vi "Create Instrument SMO Name.vi"(8 "error in (no error)":errorcluster, 11 "Instrument.Lockin":refnum<class "Instrument.Lockin.lvclass">) -> (0 "error out":errorcluster, 2 "SMO Name":string, 3 "Instrument.Lockin out":refnum<class "Instrument.Lockin.lvclass">)   [LabVIEW 2016, in "Instrument.Lockin.lvclass"]
uses:
  Instrument.Lockin.lvclass
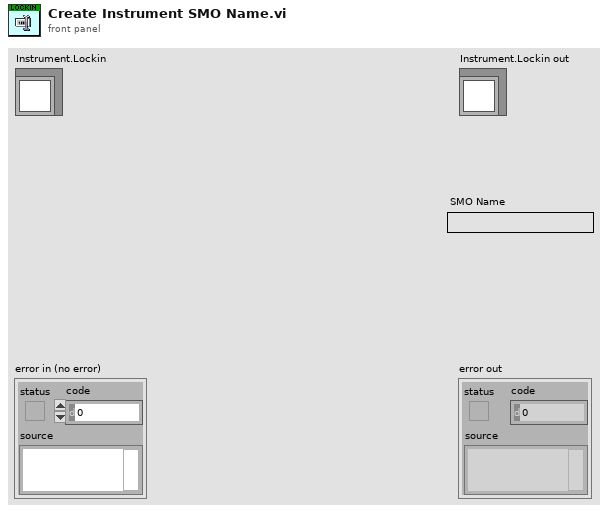
[diagram p1: front panel]
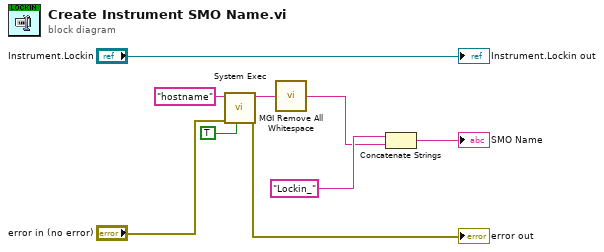
[diagram p0: block diagram]
diagram:
  n1 = call <vilib>:"System Exec.vi"("run minimized? (F)"=TRUE, "error in (no error)"="error in (no error)", "command line"="hostname") -> ("error out"=→"error out":errorcluster, "standard output"=w6:string)  [unwired: 5 in, 2 out]
  n2 = call <userlib>:"MGI Remove All Whitespace.vi"("String"=w6) -> ("Trimmed String"=w1:string)
  n3 = Concatenate Strings("Lockin_" ("SMO Name"), w1) -> (→"SMO Name":string)
  "Instrument.Lockin out" <- "Instrument.Lockin"
